vi "Password Lookup (SubVI).vi"(11 "App Data":T1) -> (2 "Boolean":bool, 3 "Disabled":T2(ring))   [LabVIEW 2021]
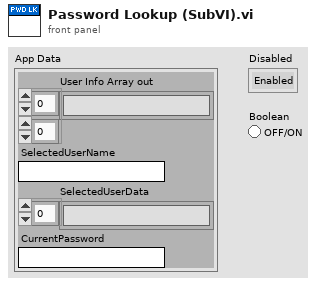
[diagram p1: front panel]
types:
  T1 = cluster{"User Info Array out":string[][], "SelectedUserName":string, "SelectedUserData":string[], "CurrentPassword":string}
  T2 = enum8{"Enabled", "Disabled", "Disabled and Grayed Out"}
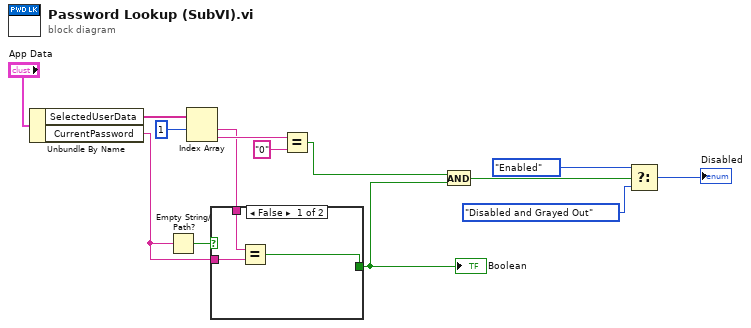
[diagram p0: block diagram]
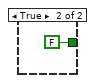
[diagram p2: hidden frame]
diagram:
  n1 = Unbundle By Name("App Data") -> ("SelectedUserData"=w4:string[], "CurrentPassword"=w2:string)
  n2 = Empty String/Path?(string/path=w2) -> (empty?=w1:bool)
  n3 = Index Array(array=w4, index #1=1 ("index")) -> (element #1=w6:string, element #2=w7:string)  [unwired: 1 in]
  n4 = case shown="False" w1 {
    tunnel: [w17 FALSE] -> w14
    tunnel: w2 -> [w16 _]
    tunnel: w6 -> [w15 _]
    frame False {
      n5 = Equal?(x=w15, y=w16) -> (x = y?=w17:bool)
    }
    frame True {
    }
  }
  "Boolean" <- w14
  n6 = Equal?(x=w7, y="0") -> (x = y?=w9:bool)
  n7 = And(x=w9, y=w14) -> (x .and. y?=w13:bool)
  n8 = Select(t=T2."Enabled" ("Disabled"), s=w13, f=T2."Disabled and Grayed Out" ("Disabled")) -> (s? t:f=→"Disabled":T2)
